vi "Set_Sections.vi"(8 "error in":errorcluster, 9 "Name":string, 10 "Path":path, 11 "Config in":refnum<class "Config.lvclass">) -> (0 "error out":errorcluster, 3 "Config out":refnum<class "Config.lvclass">)   [LabVIEW 2020, in "Config.lvclass"]
uses:
  Config.lvclass
  Config.lvclass/Config.ctl
  <vilib>/Utility/config.llb/Read Key (String).vi
  <vilib>/Utility/config.llb/NI_LVConfig.lvlib
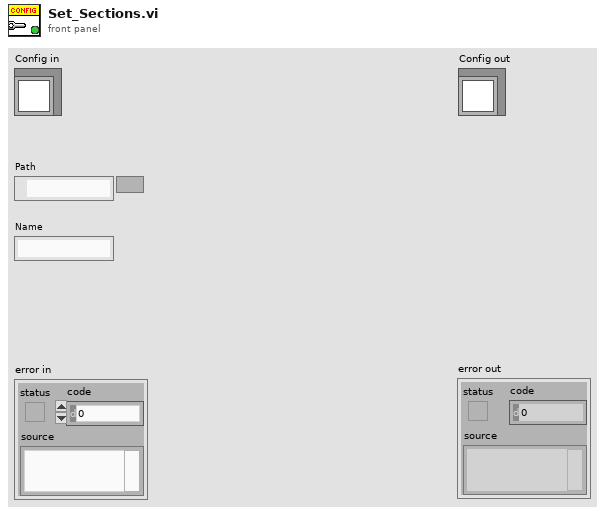
[diagram p1: front panel]
types:
  T1 = typedef "NI_LVConfig.lvlib/Config Data RefNum.ctl" = refnum<k1>
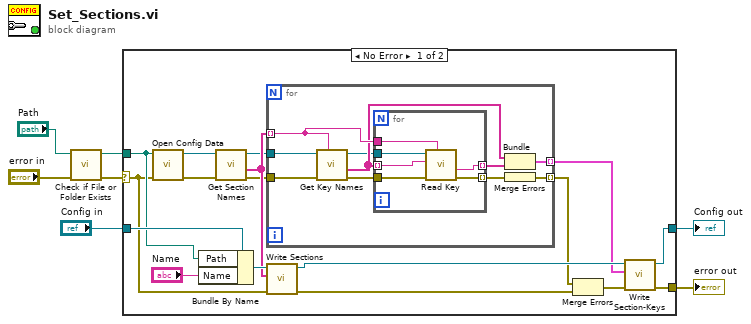
[diagram p0: block diagram]
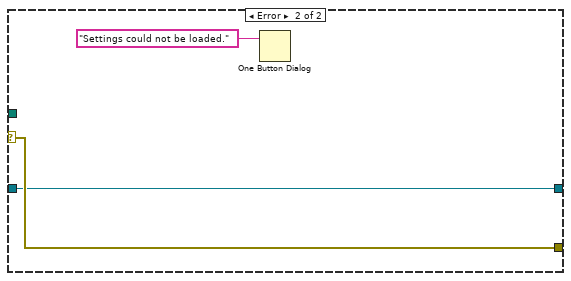
[diagram p2: hidden frame]
diagram:
  n1 = call <vilib>:"Check if File or Folder Exists.vi"("error in (no error)"="error in", "path"="Path") -> ("error out"=w4:errorcluster, "dup path"=w3:path)  [unwired: 7 in, 1 out]
  n2 = case shown="No Error" w4 {
    selector: w4 -> [w18 w43]
    tunnel: [w9 w43] -> w7
    tunnel: "Config in" -> [w24 w42]
    tunnel: w3 -> [w22 _]
    tunnel: [w13 w42] -> w2
    frame No Error {
      n3 = call <vilib>:"Open Config Data.vi"("error in (no error)"=w18, "configuration file path"=w22) -> ("error out"=w20:errorcluster, "refnum"=w21:T1)  [unwired: 7 in, 1 out]
      n4 = Bundle By Name(cluster=w24, "Path"=w22, "Name"="Name") -> (w19:refnum<class "Config.lvclass">)
      n5 = call <vilib>:"Get Section Names.vi"("error in (no error)"=w20, "refnum"=w21) -> ("error out"=w15:errorcluster, "section names"=w17:string[], "refnum out"=w16:T1)  [unwired: 7 in]
      n6 = for {
        tunnel: w17 -> [w32] mode=indexing
        tunnel: w16 -> [w34]
        tunnel: w15 -> [w33]
        tunnel: [w29] -> w10 mode=indexing
        tunnel: [w26] -> w12 mode=indexing
        n7 = call <vilib>:"Get Key Names.vi"("section"=w32, "error in (no error)"=w33, "refnum"=w34) -> ("error out"=w28:errorcluster, "key names"=w31:string[], "refnum out"=w25:T1)  [unwired: 5 in, 1 out]
        n8 = for {
          tunnel: w31 -> [w40] mode=indexing
          tunnel: w32 -> [w39]
          tunnel: [w38] -> w30 mode=indexing
          tunnel: w28 -> [w37]
          tunnel: [w36] -> w27 mode=indexing
          tunnel: w25 -> [w35]
          n9 = call-poly <vilib>:"Read Key.vi"("section"=w39, "error in (no error)"=w37, "key"=w40, "refnum"=w35) -> ("error out"=w36:errorcluster, "value"=w38:string)  [unwired: 4 in, 2 out]
        }
        n10 = Bundle("key names"=w31, w30) -> (w29:cluster{"key names":string[], string[]})  [unwired: 1 in]
        n11 = Merge Errors(w27) -> (w26:errorcluster)
      }
      n12 = call "Write Sections.vi"("error in (no error)"=w18, "Sections"=w17, "Config in"=w19) -> ("error out"=w8:errorcluster, "Config out"=w14:refnum<class "Config.lvclass">)  [unwired: 7 in]
      n13 = Merge Errors(w12, w8) -> (w11:errorcluster)
      n14 = call "Write Section-Keys.vi"("error in (no error)"=w11, "Section-Keys"=w10, "Config in"=w14) -> ("error out"=w9:errorcluster, "Config out"=w13:refnum<class "Config.lvclass">)  [unwired: 7 in]
    }
    frame Error {
      n15 = One Button Dialog(message="Settings could not be loaded.") -> ()  [unwired: 1 in, 1 out]
    }
  }
  "error out" <- w7
  "Config out" <- w2
